vi "DHE_chkStopSequence.vi"() -> (0 "error out":errorcluster)   [LabVIEW 2016]
uses:
  Common/public/vis/CMN_FVAR_action.ctl
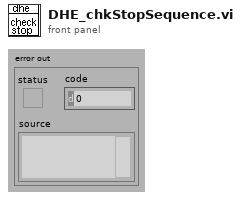
[diagram p1: front panel]
types:
  T1 = typedef "CMN_FVAR_action.ctl" = enum16{"read", "write"}
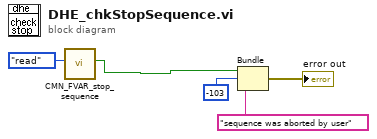
[diagram p0: block diagram]
diagram:
  n1 = call "CMN_FVAR_stop_sequence.vi"("action"=CMN_FVAR_action."read") -> ("value out"=w2:bool)  [unwired: 1 in, 8 out]
  n2 = Bundle("value out"=w2, -103, "sequence was aborted by user") -> (→"error out":cluster{"value out":bool, i32, string})  [unwired: 1 out]
